vi "Calc Cartesian Length.vi"(10 "Point 2":cluster{"x":dbl, "y":dbl, "th":dbl}, 11 "Point 1":cluster{"x":dbl, "y":dbl, "th":dbl}) -> (2 "Angle (deg)":dbl, 3 "Length (f)":dbl)   [LabVIEW 2025]
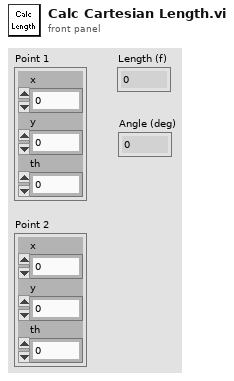
[diagram p1: front panel]
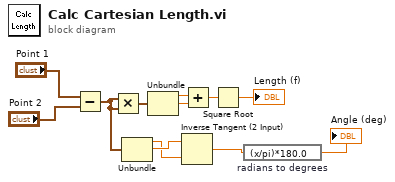
[diagram p0: block diagram]
diagram:
  n1 = Subtract(x="Point 1", y="Point 2") -> (x-y=w5:cluster{"x":dbl, "y":dbl, "th":dbl})
  n2 = Multiply(x=w5, y=w5) -> (x*y=w9:cluster{"x":dbl, "y":dbl, "th":dbl})
  n3 = Unbundle(w5) -> ("x"=w3:dbl, "y"=w4:dbl)  [unwired: 1 out]
  n4 = Unbundle(w9) -> ("x"=w8:dbl, "y"=w7:dbl)  [unwired: 1 out]
  n5 = Inverse Tangent (2 Input)(1:w3, 2:w4) -> (0:w2:dbl)
  n6 = Add(x=w8, y=w7) -> (x+y=w6:dbl)
  n7 = Square Root(x=w6) -> (sqrt(x)=→"Length (f)":dbl)
  n8 = expression code="(x/pi)*180.0" "radians to degrees"(w2) -> (→"Angle (deg)":dbl)
